vi "SetResolution.vi"(8 "error in (no error)":errorcluster, 10 "Resolution":u8 format="%.0x", 11 "CameraTesting in":refnum<class "CameraTesting.lvclass">) -> (0 "error out":errorcluster, 3 "CameraTesting out":refnum<class "CameraTesting.lvclass">)   [LabVIEW 2020, in "CameraTesting.lvlib" / "CameraTesting.lvclass"]
uses:
  CameraTesting.lvclass
  CameraTesting.lvclass/CameraTesting.ctl
  Camera/ICamera/ICamera/ICamera.lvclass
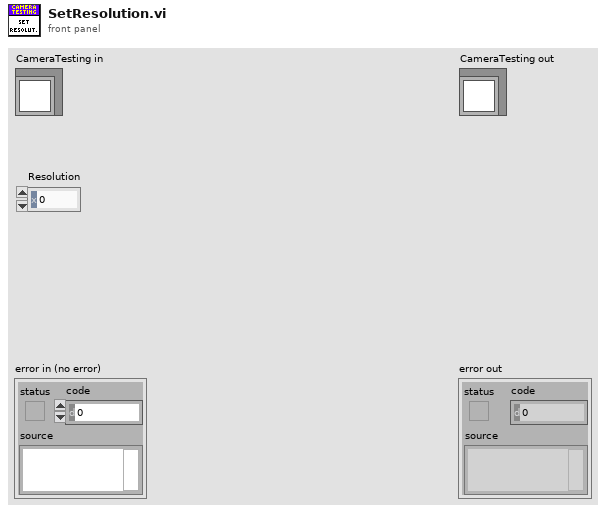
[diagram p1: front panel]
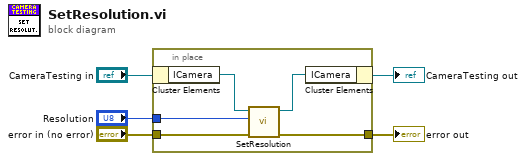
[diagram p0: block diagram]
diagram:
  n1 = in-place {
    in-place-border: "Resolution" -> [w10]
    in-place-border: "error in (no error)" -> [w9]
    in-place-border: [w8] -> w3
    n2 = in-place-cluster #1("CameraTesting in") -> ("ICamera"=w7:refnum<class "ICamera.lvclass">)
    n3 = call-dynamic "SetResolution.vi"("error in (no error)"=w9, "Resolution (hex code)"=w10, "ICamera in"=w7) -> ("error out"=w8:errorcluster, "ICamera out"=w6:refnum<class "ICamera.lvclass">)  [unwired: 7 in]
    n4 = in-place-cluster #1("ICamera"=w6) -> (→"CameraTesting out":refnum<class "CameraTesting.lvclass">)
  }
  "error out" <- w3
